vi "ReadConfig.vi"(8 "error in (no error)":errorcluster, 11 "Camera_Prime95B in":refnum<class "Camera_Prime95B.lvclass">) -> (0 "error out":errorcluster, 3 "Camera_Prime95B out":refnum<class "Camera_Prime95B.lvclass">)   [LabVIEW 2020, in "Camera_Prime95B.lvlib" / "Camera_Prime95B.lvclass"]
uses:
  Camera_Prime95B.lvclass
  Hardware Abstraction Layer/Component/Camera/Camera/Camera.lvclass
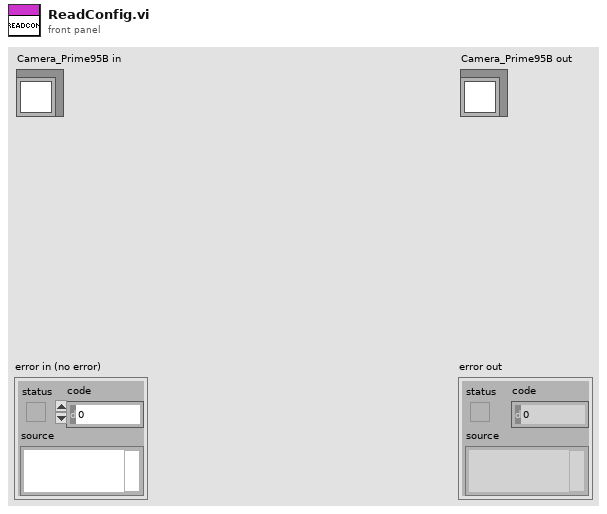
[diagram p1: front panel]
types:
  T1 = typedef "NI_LVConfig.lvlib/Config Data RefNum.ctl" = refnum<k1>
  T2 = cluster{"Values[0]":i32, "Values[1]":i32, "Values[2]":i32}
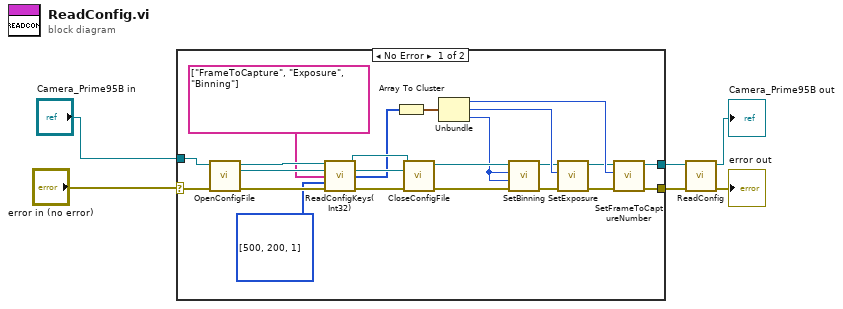
[diagram p0: block diagram]
diagram:
  n1 = case shown="No Error" "error in (no error)" {
    selector: "error in (no error)" -> [w29 w30]
    tunnel: [w16 w30] -> w1
    tunnel: [w15 w31] -> w2
    tunnel: "Camera_Prime95B in" -> [w28 w31]
    frame No Error {
      n2 = call-dynamic "OpenConfigFile.vi"("error in (no error)"=w29, "GRMActor in"=w28) -> ("error out"=w27:errorcluster, "refnum"=w23:T1, "GRMActor out"=w25:refnum<class "Camera_Prime95B.lvclass">)  [unwired: 7 in]
      n3 = call-dynamic "ReadConfigKeys(Int32).vi"("GRMActor in"=w25, "Config Refnum"=w23, "Keys"=string[] ["FrameToCapture", "Exposure", "Binning"] ("Values"), "Default"=i32[] [500, 200, 1], "error in (no error)"=w27) -> ("GRMActor out"=w21:refnum<class "Camera_Prime95B.lvclass">, "Config Refnum dup"=w20:T1, "Values"=w19:i32[], "error out"=w26:errorcluster)  [unwired: 7 in]
      n4 = Array To Cluster(array=w19) -> (cluster=w24:T2)
      n5 = call-dynamic "CloseConfigFile.vi"("error in (no error)"=w26, "refnum"=w20, "GRMActor in"=w21) -> ("error out"=w22:errorcluster, "GRMActor out"=w9:refnum<class "Camera_Prime95B.lvclass">)  [unwired: 7 in]
      n6 = Unbundle(w24) -> ("Values[0]"=w14:i32, "Values[1]"=w11:i32, "Values[2]"=w7:i32)
      n7 = call-dynamic "SetBinning.vi"("error in (no error)"=w22, "Setting.Binning.BinY"=w7, "Setting.Binning.BinX"=w7, "Camera_Prime95B in"=w9) -> ("error out"=w10:errorcluster, "Camera_Prime95B out"=w8:refnum<class "Camera_Prime95B.lvclass">)  [unwired: 6 in]
      n8 = call-dynamic "SetExposure.vi"("error in (no error)"=w10, "Setting.Exposure"=w11, "Camera_Prime95B in"=w8) -> ("error out"=w13:errorcluster, "Camera_Prime95B out"=w12:refnum<class "Camera_Prime95B.lvclass">)  [unwired: 7 in]
      n9 = call-dynamic "SetFrameToCaptureNumber.vi"("error in (no error)"=w13, "Setting.FramesToCapture"=w14, "Camera_Prime95B in"=w12) -> ("error out"=w16:errorcluster, "Camera_Prime95B out"=w15:refnum<class "Camera_Prime95B.lvclass">)  [unwired: 7 in]
    }
    frame Error {
    }
  }
  n10 = call-parent "ReadConfig.vi"("error in (no error)"=w1, "GRMActor in"=w2) -> ("error out"=→"error out":errorcluster, "GRMActor out"=→"Camera_Prime95B out":refnum<class "Camera_Prime95B.lvclass">)  [unwired: 8 in]
